vi "To Bool Tree Data.vi"(10 "Boolean":bool) -> (3 "Bool Tree Data":refnum<class "Bool.lvclass">)   [LabVIEW 2017, in "Tree API.lvlib" / "Bool.lvclass"]
doc: "Convert a Bool value to Tree Data type."
uses:
  Bool.lvclass
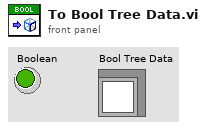
[diagram p1: front panel]
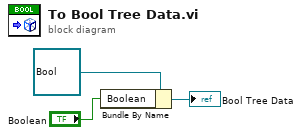
[diagram p0: block diagram]
diagram:
  n1 = Bundle By Name(cluster=refnum<class "Bool.lvclass"> refnum ("Bool in"), "Boolean"="Boolean") -> (→"Bool Tree Data":refnum<class "Bool.lvclass">)
